vi "PositionerCapture2.vi"() -> ()   [LabVIEW 2011]
doc: "CONEX - CC Virtual Front Panel:\n\nThis is a sample of an application that can be built with the LabVIEW drivers.\n\nPress HOME / ENABLE in top left of panel to put stage in Ready state for motion."
uses:
  <vilib>/userDefined/High Color/IMAQdx.ctl
  <vilib>/Platform/TimedLoop/XDataNode/timing_clust.ctl
  <vilib>/Platform/TimedLoop/XDataNode/nitl_modes.ctl
  <vilib>/Platform/TimedLoop/XDataNode/wakeup.ctl
  <vilib>/Platform/TimedLoop/XDataNode/XDataNode.xnode
  <vilib>/Platform/TimedLoop/XDataNode/XDNodeRunTimeDep.lvlib
  <vilib>/vision/driver/NI_Vision_Acquisition_Software.lvlib
panel:
  in  "component":bool
  out "amp pos":dbl
  out "Phase":bool
  out "Amp":bool
  in  "Next":bool
  out "Current noUnits":dbl caption="mm" format="%#_6f"
  in  "lambda":dbl caption="nm" format="%#_6f"
  in  "Units":string(combo)="mm"
  in  "Go0":bool
  in  "Zero position":dbl caption="mm" format="%#_6f"
  in  "Tare":bool
  out "Relative position":dbl caption="mm" format="%#_6f"
  in  "Path to save the captures":path
  out "Image":T1(plugin-control)
  in  "(1) Go to:":dbl=1.0 caption="mm"
  out "Title":string
  in  "Set Max":bool
  in  "Set Min":bool
  in  "Max":dbl
  in  "Min":dbl
  in  "Set velocity":bool
  out "Stop cycle":bool=TRUE
  out "Title 2":string
  in  "Cycle":bool
  in  "Go2":bool
  in  "Go1":bool
  in  "(2) Go to:":dbl=1.0 caption="mm"
  in  "-":bool
  in  "+":bool
  in  "Step:":dbl caption="mm" format="%#_6f"
  out "Position History":dbl(graph)=1.5
  in  "Action":bool
  out "Stop polling":bool=TRUE
  out "Controller state description":string="STATUS"
  out "Velocity MAX":dbl=0.4
  out "Controller state":string="33"
  out "Positioner error":string="0000"
  in  "Velocity:":dbl format="%#_6f"
  in  "Exit":bool=TRUE
  out "Target position":dbl
  in  "Exit":bool
  in  "Position glissière":cluster{dbl, dbl}(slide) scale=0.0..25.0
  out "Current position":dbl caption="mm" format="%#_6f"
  # "Take an image with \"Curr. Pos\" and a label as the name.\nThe label alternates between two states.\nThe position increase an step when Amp. and Phase\nis captured for both components."
  # "mm/s"
  # "mm"
  # "Limits:"
  # "mm"
  # "(1)"
  # "(2)"
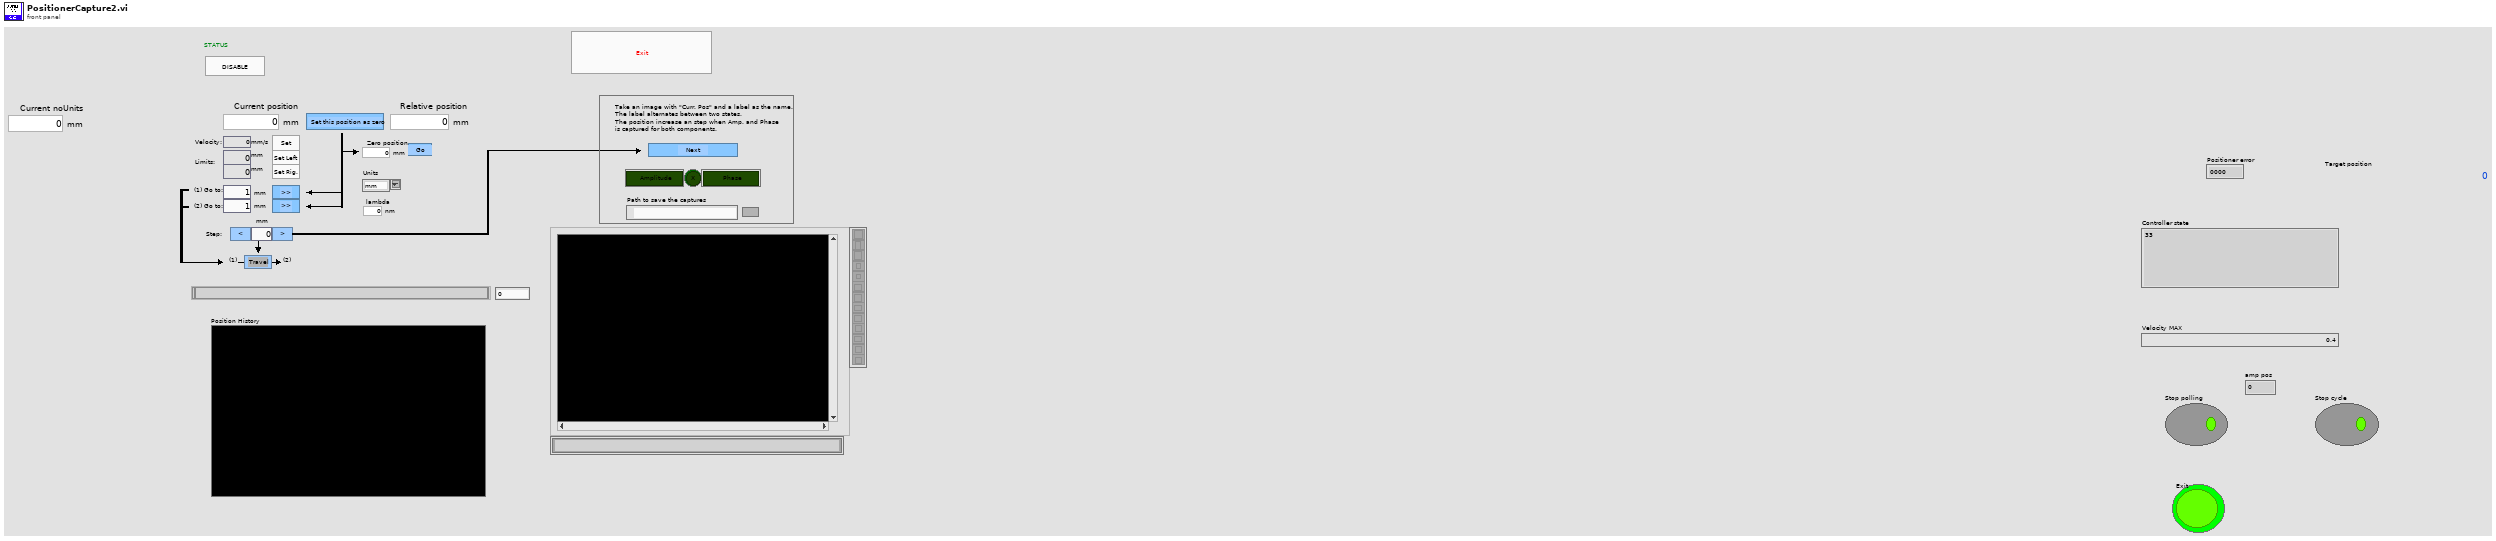
[diagram p1: front panel]
types:
  T1 = typedef "IMAQ Image.ctl" = refnum<image>
  T2 = typedef "IMAQdx.ctl" = refnum<k21>
  T3 = typedef "XDNodeRunTimeDep.lvlib/timing_clust.ctl" = cluster{"Expected End [f-1]":u64, "Actual End [f-1]":u64, "Finished Late? [f-1]":bool, "Expected End [i-1]":u64, "Actual End [i-1]":u64, "Finished Late? [i-1]":bool, "Expected Start [i]":u64, "Actual Start [i]":u64, "Expected Start [f]":u64, "Actual Start [f]":u64, "Source Name":string, "Structure Name":string, "Period":i64, "Deadline":i64, "Offset":i64, "Start":i64, "Priority":i32, "Timeout":i32, "Mode":T4, "Wakeup Reason":T5, "Error":errorcluster, "Source Type":string, "Secondary Source Type":string, "Global End Time":u64, "Global Start Time":u64, "Frame Duration":u64, "Iteration Duration":u64, "Assigned CPU":i32, "I/O Scan Engine Mode":u32}
  T4 = typedef "XDNodeRunTimeDep.lvlib/nitl_modes.ctl" = enum32{"No Change", "Process missed periods, maintain original phase", "Discard missed periods, maintain original phase", "Process missed periods, ignore original phase", "Discard missed periods, ignore original phase"}
  T5 = typedef "XDNodeRunTimeDep.lvlib/wakeup.ctl" = enum32{"Normal", "Aborted", "Asynchronous wakeup", "Timing source error", "Timed loop error", "Timeout"}
  T6 = cluster{"VISA resource name":refnum<visa-resource-name>, "Device name":string, "Controller address":i32, "error":errorcluster}
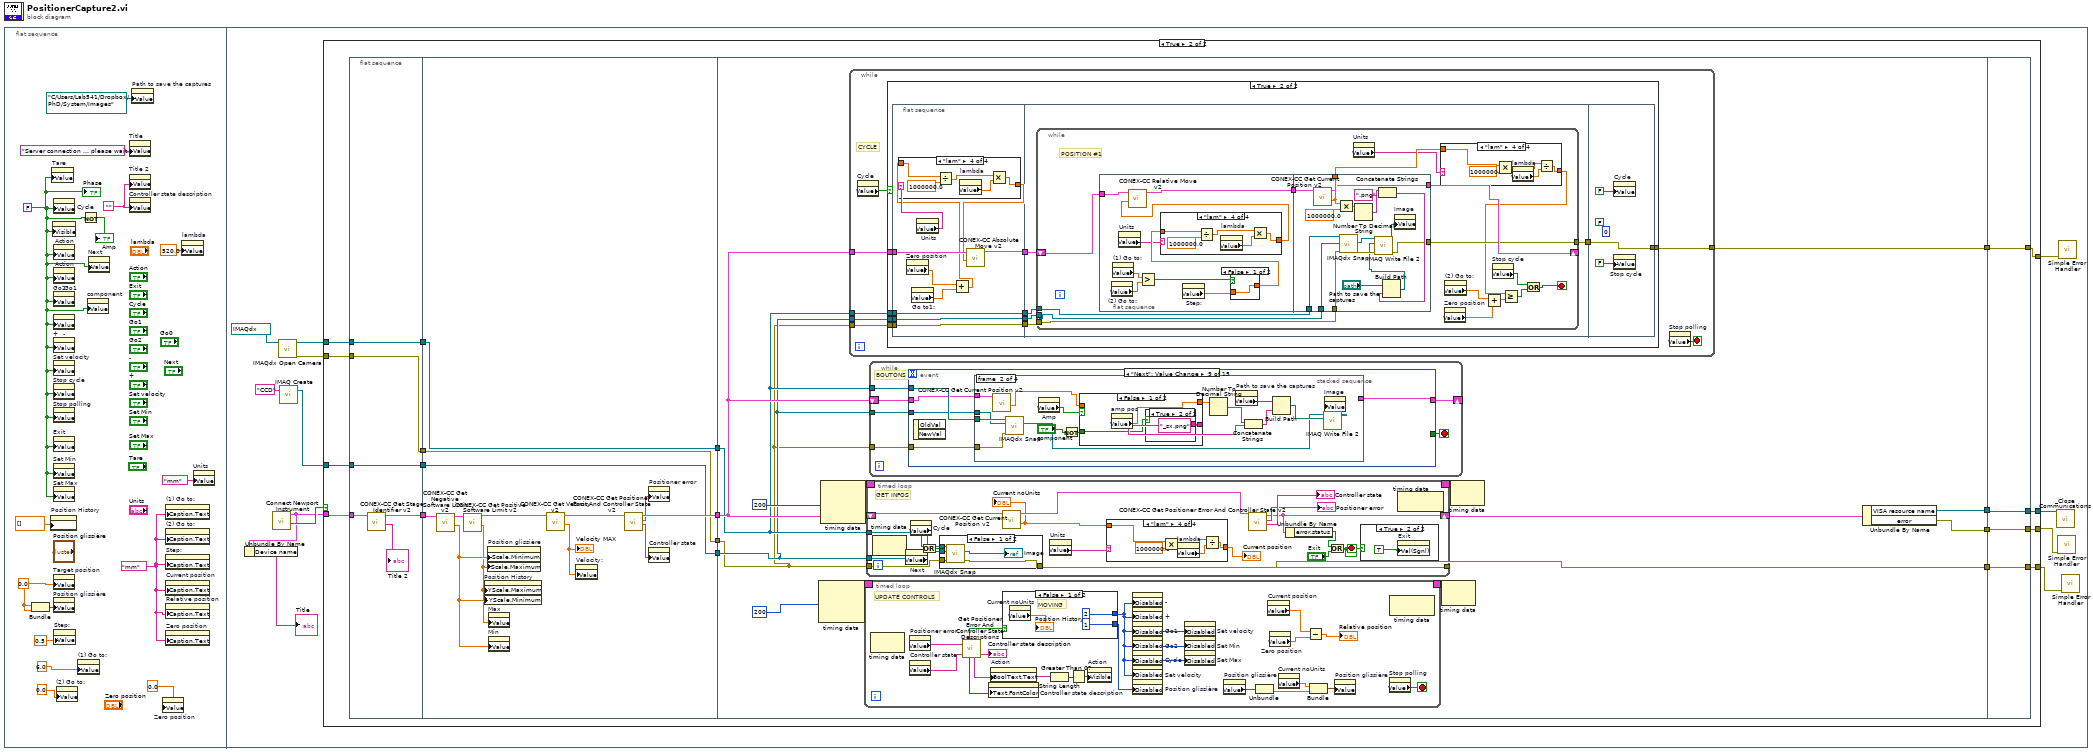
[diagram p0: block diagram]
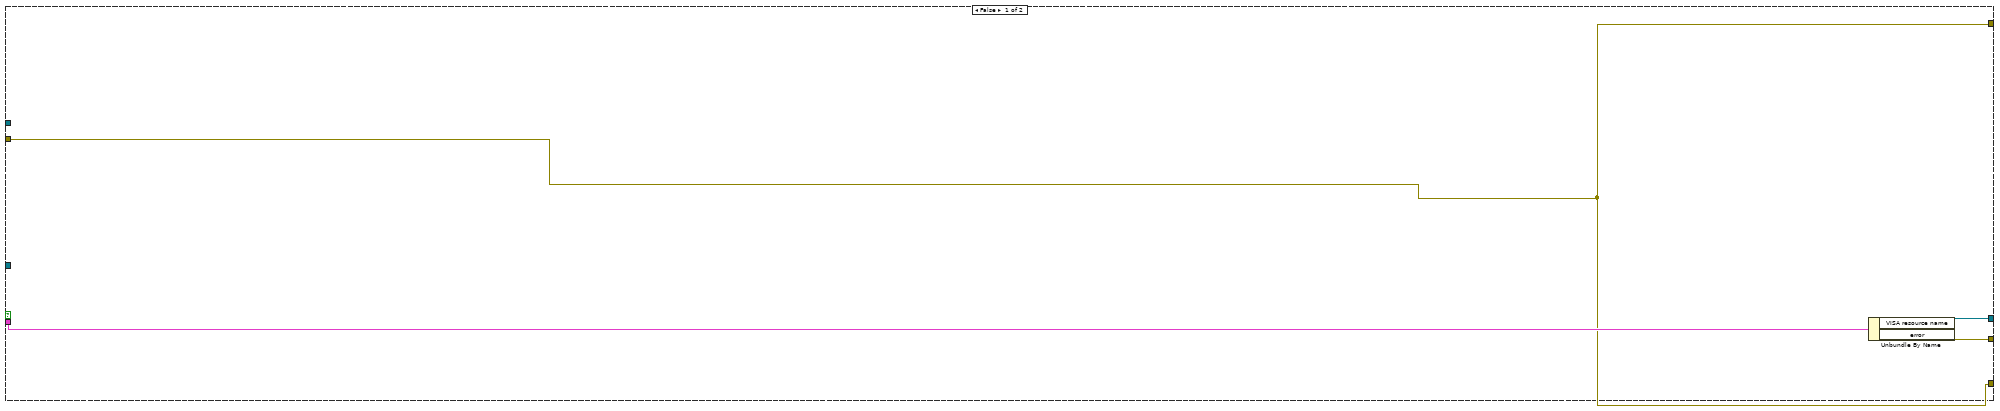
[diagram p2: hidden frame]
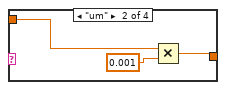
[diagram p5: hidden frame]
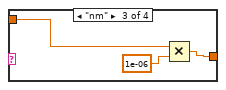
[diagram p6: hidden frame]
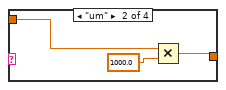
[diagram p8: hidden frame]
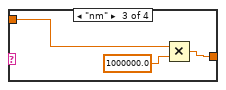
[diagram p9: hidden frame]
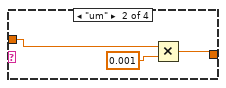
[diagram p11: hidden frame]
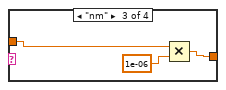
[diagram p12: hidden frame]
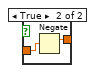
[diagram p13: hidden frame]
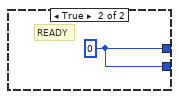
[diagram p14: hidden frame]
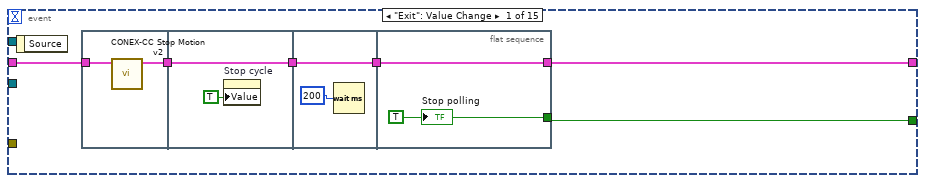
[diagram p15: hidden frame]
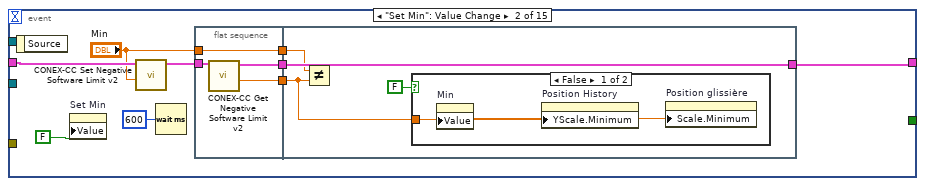
[diagram p16: hidden frame]
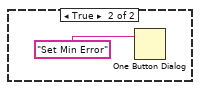
[diagram p17: hidden frame]
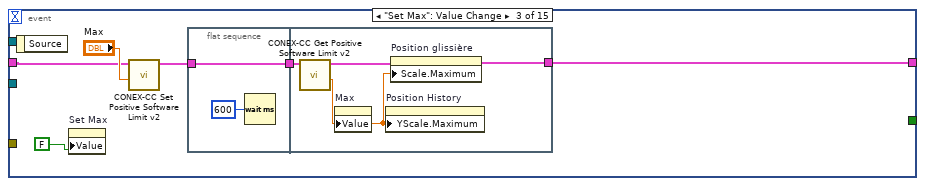
[diagram p18: hidden frame]
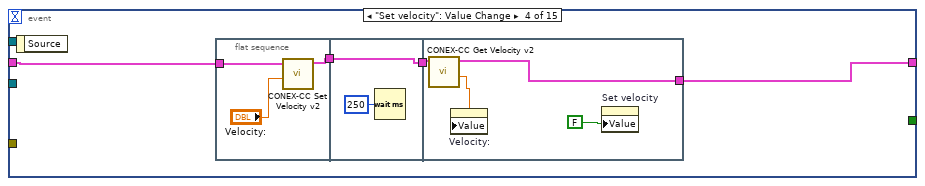
[diagram p19: hidden frame]
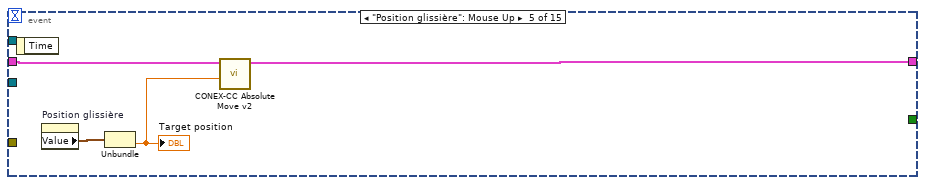
[diagram p20: hidden frame]
diagram:
  n1 = flat-sequence {
    frame #0 {
      w5 = "mm" ("Units")
      w1 = FALSE
      w14 = 0.0
      w13 = ""
      n2 = Bundle(w14, w14) -> (w15:cluster{dbl, dbl})  [unwired: 1 out]
      n3 = property on="Position History" class="WFChart (strict)"("History Data"=dbl[] [] ("Données d'historique")) -> ()  [unwired: 2 in, 2 out]
      n4 = property on="Tare" class="Bool (strict)"("Value"=w1) -> ()  [unwired: 2 in, 2 out]
      n5 = property on="Action" class="Bool (strict)"("Visible"=w1) -> ()  [unwired: 2 in, 2 out]
      n6 = property on="Cycle" class="Bool (strict)"("Value"=w1) -> ()  [unwired: 2 in, 2 out]
      n7 = property on="Action" class="Bool (strict)"("Value"=w1) -> ()  [unwired: 2 in, 2 out]
      n8 = property on="Go1" class="Bool (strict)"("Value"=w1) -> ()  [unwired: 2 in, 2 out]
      n9 = property on="Go2" class="Bool (strict)"("Value"=w1) -> ()  [unwired: 2 in, 2 out]
      n10 = property on="-" class="Bool (strict)"("Value"=w1) -> ()  [unwired: 2 in, 2 out]
      n11 = property on="+" class="Bool (strict)"("Value"=w1) -> ()  [unwired: 2 in, 2 out]
      n12 = property on="Set velocity" class="Bool (strict)"("Value"=w1) -> ()  [unwired: 2 in, 2 out]
      n13 = property on="Stop cycle" class="Bool (strict)"("Value"=w1) -> ()  [unwired: 2 in, 2 out]
      n14 = property on="Stop polling" class="Bool (strict)"("Value"=w1) -> ()  [unwired: 2 in, 2 out]
      n15 = property on="Exit" class="Bool (strict)"("Value"=w1) -> ()  [unwired: 2 in, 2 out]
      n16 = property on="Set Min" class="Bool (strict)"("Value"=w1) -> ()  [unwired: 2 in, 2 out]
      n17 = property on="Set Max" class="Bool (strict)"("Value"=w1) -> ()  [unwired: 2 in, 2 out]
      n18 = property on="Target position" class="DigNum (strict)"("Value"=w14) -> ()  [unwired: 2 in, 2 out]
      n19 = property on="Position glissière" class="Slide (strict)"("Value"=w15) -> ()  [unwired: 2 in, 2 out]
      n20 = property on="Step:" class="DigNum (strict)"("Value"=0.5 ("Step")) -> ()  [unwired: 2 in, 2 out]
      n21 = property on="(2) Go to:" class="DigNum (strict)"("Value"=0.0 ("Abs. Move 2")) -> ()  [unwired: 2 in, 2 out]
      n22 = property on="(1) Go to:" class="DigNum (strict)"("Value"=6.0 ("Abs. Move 1")) -> ()  [unwired: 2 in, 2 out]
      n23 = Not(x=w1) -> (.not. x?=→"Amp":bool)
      n24 = property on="component" class="Bool (strict)"("Value"=w1) -> ()  [unwired: 2 in, 2 out]
      n25 = property on="Next" class="Bool (strict)"("Value"=w1) -> ()  [unwired: 2 in, 2 out]
      n26 = property on="Title" class="Str"("Value"="Server connection ... please wait." ("Title")) -> ()  [unwired: 2 in, 2 out]
      n27 = property on="Title 2" class="Str"("Value"=w13) -> ()  [unwired: 2 in, 2 out]
      n28 = property on="Controller state description" class="Str"("Value"=w13) -> ()  [unwired: 2 in, 2 out]
      n29 = property on="Path to save the captures" class="Path"("Value"=path "C:/Users/Lab541/Dropbox/PhD/System/Images" ("Path to save the captures")) -> ()  [unwired: 2 in, 2 out]
      n30 = property on="Zero position" class="DigNum (strict)"("Value"=0.0 ("Zero position")) -> ()  [unwired: 2 in, 2 out]
      n31 = property on="(1) Go to:" class="DigNum (strict)"("Caption.Text"=w5) -> ()  [unwired: 2 in, 2 out]
      n32 = property on="(2) Go to:" class="DigNum (strict)"("Caption.Text"=w5) -> ()  [unwired: 2 in, 2 out]
      n33 = property on="Step:" class="DigNum (strict)"("Caption.Text"=w5) -> ()  [unwired: 2 in, 2 out]
      n34 = property on="Current position" class="DigNum (strict)"("Caption.Text"=w5) -> ()  [unwired: 2 in, 2 out]
      n35 = property on="Relative position" class="DigNum (strict)"("Caption.Text"=w5) -> ()  [unwired: 2 in, 2 out]
      n36 = property on="Zero position" class="DigNum (strict)"("Caption.Text"=w5) -> ()  [unwired: 2 in, 2 out]
      n37 = property on="lambda" class="DigNum (strict)"("Value"=520.0 ("lambda")) -> ()  [unwired: 2 in, 2 out]
      n38 = property on="Units" class="CmbBox"("Value"="mm" ("Units")) -> ()  [unwired: 2 in, 2 out]
      "Phase" <- w1
    }
    frame #1 {
      n39 = call <userlib>:"Connect Newport Instrument.vi"() -> ("Connected"=w25:bool, "Device Connection Cluster"=w24:T6)  [unwired: 7 in, 3 out]
      n40 = Unbundle By Name(w24) -> ("Device name"=→"Title":string)
      n41 = call <vilib>:"IMAQdx Open Camera.vi"("Session In"=T2 "Paraxial") -> ("error out"=w18:errorcluster, "Session Out"=w20:T2)  [unwired: 9 in]
      n42 = call "IMAQ Create"("Image Name"="CCD") -> ("New Image"=w19:T1)  [unwired: 4 in, 1 out]
      n43 = case shown="True" w25 {
        tunnel: [w30 w51] -> w27
        tunnel: w24 -> [w31 w49]
        tunnel: [w29 w45] -> w23
        tunnel: w20 -> [_ w43]
        tunnel: w19 -> [_ w40]
        tunnel: w18 -> [w28 w37]
        tunnel: [w28 w34] -> w17
        tunnel: [w28 w32] -> w16
        frame False {
          n44 = Unbundle By Name(w31) -> ("VISA resource name"=w29:refnum<visa-resource-name>, "error"=w30:errorcluster)
        }
        frame True {
          n45 = flat-sequence {
            tunnel: w49 -> [w57]
            tunnel: [w55] -> w48
            tunnel: [w54] -> w44
            tunnel: w43 -> [w54]
            tunnel: [w53] -> w41
            tunnel: w40 -> [w53]
            tunnel: [w52] -> w38
            tunnel: w37 -> [w52]
            tunnel: [w67] -> w50
            tunnel: w48 -> [w64]
            tunnel: w44 -> [w60]
            tunnel: [w60] -> w42
            tunnel: w41 -> [w59]
            tunnel: [w59] -> w39
            tunnel: w38 -> [w58]
            tunnel: [w58] -> w36
            tunnel: w50 -> [w76]
            tunnel: [w78] -> w47
            tunnel: [w77] -> w46
            tunnel: w42 -> [w73]
            tunnel: w39 -> [w72]
            tunnel: w36 -> [w71]
            tunnel: [w75] -> w35
            tunnel: [w74] -> w33
            tunnel: [w543] -> w51
            tunnel: w47 -> [w542]
            tunnel: w46 -> [w543]
            tunnel: [w542] -> w45
            tunnel: [w541] -> w34
            tunnel: w35 -> [w541]
            tunnel: [w540] -> w32
            tunnel: w33 -> [w540]
            frame #0 {
              n46 = call <userlib>:"CONEX-CC Get Stage Identifier v2.vi"("Connection Cluster in"=w57) -> ("Identifier"=→"Title 2":string, "Connection Cluster out"=w55:T6)  [unwired: 9 in]
            }
            frame #1 {
              n47 = call <userlib>:"CONEX-CC Get Negative Software Limit v2.vi"("Connection Cluster in"=w64) -> ("Left limit"=w69:dbl, "Connection Cluster out"=w63:T6)  [unwired: 9 in]
              n48 = call <userlib>:"CONEX-CC Get Positive Software Limit v2.vi"("Connection Cluster in"=w63) -> ("Right limit"=w68:dbl, "Connection Cluster out"=w62:T6)  [unwired: 9 in]
              n49 = property on="Position History" class="WFChart (strict)"("YScale.Maximum"=w68, "YScale.Minimum"=w69) -> ()  [unwired: 2 in, 2 out]
              n50 = property on="Position glissière" class="Slide (strict)"("Scale.Minimum"=w69, "Scale.Maximum"=w68) -> ()  [unwired: 2 in, 2 out]
              n51 = property on="Max" class="DigNum (strict)"("Value"=w68) -> ()  [unwired: 2 in, 2 out]
              n52 = property on="Min" class="DigNum (strict)"("Value"=w69) -> ()  [unwired: 2 in, 2 out]
              n53 = call <userlib>:"CONEX-CC Get Velocity v2.vi"("Connection Cluster in"=w62) -> ("Velocity"=w70:dbl, "Connection Cluster out"=w61:T6)  [unwired: 8 in, 1 out]
              "Velocity MAX" <- w70
              n54 = property on="Velocity:" class="DigNum (strict)"("Value"=w70) -> ()  [unwired: 2 in, 2 out]
              n55 = call <userlib>:"CONEX-CC Get Positioner Error And Controller State v2.vi"("Connection Cluster in"=w61) -> ("Controller state"=w65:string, "Positioner error"=w66:string, "Connection Cluster out"=w67:T6)  [unwired: 8 in]
              n56 = property on="Positioner error" class="Str"("Value"=w66) -> ()  [unwired: 2 in, 2 out]
              n57 = property on="Controller state" class="Str"("Value"=w65) -> ()  [unwired: 2 in, 2 out]
            }
            frame #2 {
              n58 = node-c288(i64 200 ("Période")) -> (w83:T3)  [unwired: 1 in, 1 out]
              n59 = node-c288(i64 200 ("Période")) -> (w85:T3)  [unwired: 1 in, 1 out]
              n60 = while {
                tunnel: w76 -> [w92]
                tunnel: w73 -> [w89]
                tunnel: w72 -> [w88]
                tunnel: w71 -> [w87]
                tunnel: [w86] -> w74
                stop <- w91 stop-if-true
                # "CYCLE"
                n61 = property on="Cycle" class="Bool (strict)"() -> ("Value"=w90:bool)  [unwired: 2 in, 2 out]
                n62 = case shown="True" w90 {
                  tunnel: w92 -> [_ w103]
                  tunnel: w89 -> [_ w100]
                  tunnel: w88 -> [_ w98]
                  tunnel: w87 -> [w93 w96]
                  tunnel: [w93 w95] -> w86
                  frame False {
                  }
                  frame True {
                    n63 = flat-sequence {
                      tunnel: w103 -> [w113]
                      tunnel: [w112] -> w102
                      tunnel: [w111] -> w101
                      tunnel: w100 -> [w111]
                      tunnel: [w110] -> w99
                      tunnel: w98 -> [w110]
                      tunnel: [w109] -> w97
                      tunnel: w96 -> [w109]
                      tunnel: w102 -> [w130]
                      tunnel: w101 -> [w129]
                      tunnel: w99 -> [w128]
                      tunnel: w97 -> [w127]
                      tunnel: [w126] -> w94
                      tunnel: [w200] -> w95
                      tunnel: w94 -> [w200]
                      frame #0 {
                        n64 = property on="Zero position" class="DigNum (strict)"() -> ("Value"=w104:dbl)  [unwired: 2 in, 2 out]
                        n65 = property on="Go to1:" class="DigNum (strict)"() -> ("Value"=w106:dbl)  [unwired: 2 in, 2 out]
                        n66 = property on="Units" class="CmbBox"() -> ("Value"=w107:string)  [unwired: 2 in, 2 out]
                        n67 = Add(x=w104, y=w106) -> (x+y=w105:dbl)
                        n68 = case shown="\"lam\"" w107 {
                          tunnel: [w114 w115 w118 w121] -> w108
                          tunnel: w105 -> [w114 w116 w119 w125]
                          frame "mm", Default {
                          }
                          frame "um" {
                            n69 = Multiply(x=w116, y=0.001) -> (x*y=w115:dbl)
                          }
                          frame "nm" {
                            n70 = Multiply(x=w119, y=1e-06) -> (x*y=w118:dbl)
                          }
                          frame "lam" {
                            n71 = Divide(x=w125, y=1000000.0) -> (x/y=w123:dbl)
                            n72 = property on="lambda" class="DigNum (strict)"() -> ("Value"=w122:dbl)  [unwired: 2 in, 2 out]
                            n73 = Multiply(x=w123, y=w122) -> (x*y=w121:dbl)
                          }
                        }
                        n74 = call <userlib>:"CONEX-CC Absolute Move v2.vi"("Target position"=w108, "Connection Cluster in"=w113) -> ("Connection Cluster out"=w112:T6)  [unwired: 5 in, 2 out]
                      }
                      frame #1 {
                        n75 = while {
                          shift-right: [w139] -> _
                          shift-left: w130 -> [w145]
                          tunnel: w129 -> [w141]
                          tunnel: w128 -> [w140]
                          tunnel: w127 -> [w142]
                          tunnel: [w138] -> w126
                          stop <- w146 stop-if-true
                          # "POSITION #1"
                          n76 = flat-sequence {
                            tunnel: w145 -> [w167]
                            tunnel: [w166] -> w137
                            tunnel: w141 -> [w199]
                            tunnel: w140 -> [w198]
                            tunnel: w142 -> [w197]
                            tunnel: w137 -> [w193]
                            tunnel: [w185] -> w136
                            tunnel: [w184] -> w139
                            tunnel: [w183] -> w138
                            frame #0 {
                              n77 = property on="(2) Go to:" class="DigNum (strict)"() -> ("Value"=w165:dbl)  [unwired: 2 in, 2 out]
                              n78 = property on="(1) Go to:" class="DigNum (strict)"() -> ("Value"=w164:dbl)  [unwired: 2 in, 2 out]
                              n79 = property on="Units" class="CmbBox"() -> ("Value"=w159:string)  [unwired: 2 in, 2 out]
                              n80 = Greater?(x=w164, y=w165) -> (0:w163:bool)
                              n81 = property on="Step:" class="DigNum (strict)"() -> ("Value"=w162:dbl)  [unwired: 2 in, 2 out]
                              n82 = case shown="False" w163 {
                                tunnel: [w180 w181] -> w161
                                tunnel: w162 -> [w180 w182]
                                frame False {
                                }
                                frame True {
                                n83 = Negate(x=w182) -> (-x=w181:dbl)
                                }
                              }
                              n84 = case shown="\"lam\"" w159 {
                                tunnel: [w168 w170 w173 w176] -> w160
                                tunnel: w161 -> [w168 w169 w172 w175]
                                frame "mm", Default {
                                }
                                frame "um" {
                                n85 = Multiply(x=w169, y=0.001) -> (x*y=w170:dbl)
                                }
                                frame "nm" {
                                n86 = Multiply(x=w172, y=1e-06) -> (x*y=w173:dbl)
                                }
                                frame "lam" {
                                n87 = Divide(x=w175, y=1000000.0) -> (x/y=w178:dbl)
                                n88 = property on="lambda" class="DigNum (strict)"() -> ("Value"=w177:dbl)  [unwired: 2 in, 2 out]
                                n89 = Multiply(x=w178, y=w177) -> (x*y=w176:dbl)
                                }
                              }
                              n90 = call <userlib>:"CONEX-CC Relative Move v2.vi"("Relative displacement"=w160, "Connection Cluster in"=w167) -> ("Connection Cluster out"=w166:T6)  [unwired: 9 in]
                            }
                            frame #1 {
                              n91 = call <userlib>:"CONEX-CC Get Current Position v2.vi"("Connection Cluster in"=w193) -> ("Current position"=w185:dbl, "Connection Cluster out"=w184:T6)  [unwired: 8 in, 1 out]
                              n92 = Multiply(x=w185, y=1000000.0) -> (x*y=w189:dbl)
                              n93 = call <vilib>:"IMAQdx Snap.vi"("error in"=w197, "Image In"=w198, "Session In"=w199) -> ("error out"=w195:errorcluster, "Image Out"=w196:T1)  [unwired: 6 in, 1 out]
                              n94 = Number To Decimal String(number=w189) -> (decimal integer string=w188:string)  [unwired: 1 in]
                              n95 = Concatenate Strings(w188, ".png" ("string")) -> (w186:string)
                              n96 = Build Path(base path="Path to save the captures", name or relative path=w186) -> (appended path=w190:path)
                              n97 = call-poly "IMAQ Write File 2"("error in (no error)"=w195, "File Path"=w190, "Image"=w196) -> ("error out"=w183:errorcluster, "Image Out (duplicate)"=w194:T1)  [unwired: 7 in]
                              n98 = property on="Image" class="ImageControl"("Value"=w194) -> ()  [unwired: 2 in, 2 out]
                            }
                          }
                          n99 = property on="Units" class="CmbBox"() -> ("Value"=w134:string)  [unwired: 2 in, 2 out]
                          n100 = case shown="\"lam\"" w134 {
                            tunnel: [w147 w148 w151 w154] -> w135
                            tunnel: w136 -> [w147 w149 w152 w155]
                            frame "mm", Default {
                            }
                            frame "um" {
                              n101 = Multiply(x=w149, y=1000.0) -> (x*y=w148:dbl)
                            }
                            frame "nm" {
                              n102 = Multiply(x=w152, y=1000000.0) -> (x*y=w151:dbl)
                            }
                            frame "lam" {
                              n103 = Multiply(x=w155, y=1000000.0) -> (x*y=w158:dbl)
                              n104 = property on="lambda" class="DigNum (strict)"() -> ("Value"=w156:dbl)  [unwired: 2 in, 2 out]
                              n105 = Divide(x=w158, y=w156) -> (x/y=w154:dbl)
                            }
                          }
                          n106 = property on="Zero position" class="DigNum (strict)"() -> ("Value"=w131:dbl)  [unwired: 2 in, 2 out]
                          n107 = property on="(2) Go to:" class="DigNum (strict)"() -> ("Value"=w132:dbl)  [unwired: 2 in, 2 out]
                          n108 = Add(x=w132, y=w131) -> (x+y=w133:dbl)
                          n109 = property on="Stop cycle" class="Bool (strict)"() -> ("Value"=w143:bool)  [unwired: 2 in, 2 out]
                          n110 = Greater Or Equal?(x=w135, y=w133) -> (x >= y?=w144:bool)
                          n111 = Or(x=w143, y=w144) -> (x .or. y?=w146:bool)
                        }
                      }
                      frame #2 {
                        (unwired) 0 ("counter")
                        (unwired) FALSE ("Visible")
                        n112 = property on="Cycle" class="Bool (strict)"("Value"=FALSE ("Cycle")) -> ()  [unwired: 2 in, 2 out]
                        n113 = property on="Stop cycle" class="Bool (strict)"("Value"=FALSE ("Cycle")) -> ()  [unwired: 2 in, 2 out]
                      }
                    }
                  }
                }
                n114 = property on="Stop polling" class="Bool (strict)"() -> ("Value"=w91:bool)  [unwired: 2 in, 2 out]
              }
              n115 = timed-loop {
                timing: w83 -> [_]
                timing-out: [_] -> w82
                stop <- w211 stop-if-true
                # "UPDATE CONTROLS"
                n116 = node-c288() -> ()  [unwired: 2 out]
                n117 = property on="Positioner error" class="Str"() -> ("Value"=w220:string)  [unwired: 2 in, 2 out]
                n118 = property on="Controller state" class="Str"() -> ("Value"=w219:string)  [unwired: 2 in, 2 out]
                n119 = call <userlib>:"Get Positioner Error And Controller State Descriptions.vi"("Controller state"=w219, "Positioner error"=w220) -> ("Color"=w217:u32, "Action name"=w216:string, "Controller state description"=→"Controller state description":string, "IsReady?"=w213:bool)  [unwired: 2 out]
                n120 = property on="Controller state description" class="Str"("Text.FontColor"=w217) -> ()  [unwired: 2 in, 2 out]
                n121 = property on="Action" class="Bool (strict)"("BoolText.Text"=w216) -> ()  [unwired: 2 in, 2 out]
                n122 = case shown="False" w213 {
                  tunnel: [u8 2 w224] -> w210
                  tunnel: [u8 1 w224] -> w212
                  frame False {
                    # "MOVING"
                    n123 = property on="Current noUnits" class="DigNum (strict)"() -> ("Value"=→"Position History":dbl)  [unwired: 2 in, 2 out]
                  }
                  frame True {
                    w224 = u8 0
                    # "READY"
                  }
                }
                n124 = String Length(string=w216) -> (length=w215:i32)
                n125 = Greater Than 0?(x=w215) -> (x > 0?=w214:bool)
                n126 = property on="Action" class="Bool (strict)"("Visible"=w214) -> ()  [unwired: 2 in, 2 out]
                n127 = property on="-" class="Bool (strict)"("Disabled"=w210) -> ()  [unwired: 2 in, 2 out]
                n128 = property on="+" class="Bool (strict)"("Disabled"=w210) -> ()  [unwired: 2 in, 2 out]
                n129 = property on="Go1" class="Bool (strict)"("Disabled"=w210) -> ()  [unwired: 2 in, 2 out]
                n130 = property on="Go2" class="Bool (strict)"("Disabled"=w210) -> ()  [unwired: 2 in, 2 out]
                n131 = property on="Cycle" class="Bool (strict)"("Disabled"=w210) -> ()  [unwired: 2 in, 2 out]
                n132 = property on="Set velocity" class="Bool (strict)"("Disabled"=w210) -> ()  [unwired: 2 in, 2 out]
                n133 = property on="Position glissière" class="Slide (strict)"("Disabled"=w212) -> ()  [unwired: 2 in, 2 out]
                n134 = property on="Set velocity" class="Bool (strict)"("Disabled"=w210) -> ()  [unwired: 2 in, 2 out]
                n135 = property on="Set Min" class="Bool (strict)"("Disabled"=w210) -> ()  [unwired: 2 in, 2 out]
                n136 = property on="Set Max" class="Bool (strict)"("Disabled"=w210) -> ()  [unwired: 2 in, 2 out]
                n137 = property on="Position glissière" class="Slide (strict)"() -> ("Value"=w208:cluster{dbl, dbl})  [unwired: 2 in, 2 out]
                n138 = Unbundle(w208) -> (w207:dbl)  [unwired: 1 out]
                n139 = property on="Current position" class="DigNum (strict)"() -> ("Value"=w203:dbl)  [unwired: 2 in, 2 out]
                n140 = property on="Zero position" class="DigNum (strict)"() -> ("Value"=w204:dbl)  [unwired: 2 in, 2 out]
                n141 = property on="Current noUnits" class="DigNum (strict)"() -> ("Value"=w205:dbl)  [unwired: 2 in, 2 out]
                n142 = Subtract(x=w203, y=w204) -> (x-y=→"Relative position":dbl)
                n143 = Bundle("Value"=w205, w207) -> (w209:cluster{"Value":dbl, dbl})  [unwired: 1 out]
                n144 = property on="Position glissière" class="Slide (strict)"("Value"=w209) -> ()  [unwired: 2 in, 2 out]
                n145 = node-c288() -> ()  [unwired: 2 out]
                n146 = property on="Stop polling" class="Bool (strict)"() -> ("Value"=w211:bool)  [unwired: 2 in, 2 out]
              }
              n147 = timed-loop {
                timing: w85 -> [_]
                timing-out: [_] -> w84
                shift-right: [w505] -> w79
                shift-left: w76 -> [w514]
                tunnel: w73 -> [w513]
                tunnel: w72 -> [w512]
                tunnel: w71 -> [w511]
                tunnel: [w510] -> w75
                stop <- w508 stop-if-true
                # "GET INFOS"
                n148 = node-c288() -> ()  [unwired: 2 out]
                n149 = property on="Next" class="Bool (strict)"() -> ("Value"=w497:bool)  [unwired: 2 in, 2 out]
                n150 = property on="Cycle" class="Bool (strict)"() -> ("Value"=w499:bool)  [unwired: 2 in, 2 out]
                n151 = Or(x=w499, y=w497) -> (x .or. y?=w498:bool)
                n152 = case shown="False" w498 {
                  tunnel: w513 -> [w531 _]
                  tunnel: w512 -> [w530 _]
                  tunnel: w511 -> [w529 w532]
                  tunnel: [w527 w532] -> w510
                  frame False {
                    n153 = call <vilib>:"IMAQdx Snap.vi"("error in"=w529, "Image In"=w530, "Session In"=w531) -> ("error out"=w527:errorcluster, "Image Out"=→"Image":T1)  [unwired: 6 in, 1 out]
                  }
                  frame True {
                  }
                }
                n154 = call <userlib>:"CONEX-CC Get Current Position v2.vi"("Connection Cluster in"=w514) -> ("Current position"=w501:dbl, "Connection Cluster out"=w502:T6)  [unwired: 8 in, 1 out]
                "Current noUnits" <- w501
                n155 = property on="Units" class="CmbBox"() -> ("Value"=w500:string)  [unwired: 2 in, 2 out]
                n156 = case shown="\"lam\"" w500 {
                  tunnel: [w515 w516 w519 w522] -> w504
                  tunnel: w501 -> [w515 w517 w520 w523]
                  frame "mm", Default {
                  }
                  frame "um" {
                    n157 = Multiply(x=w517, y=1000.0) -> (x*y=w516:dbl)
                  }
                  frame "nm" {
                    n158 = Multiply(x=w520, y=1000000.0) -> (x*y=w519:dbl)
                  }
                  frame "lam" {
                    n159 = Multiply(x=w523, y=1000000.0) -> (x*y=w526:dbl)
                    n160 = property on="lambda" class="DigNum (strict)"() -> ("Value"=w524:dbl)  [unwired: 2 in, 2 out]
                    n161 = Divide(x=w526, y=w524) -> (x/y=w522:dbl)
                  }
                }
                "Current position" <- w504
                n162 = call <userlib>:"CONEX-CC Get Positioner Error And Controller State v2.vi"("Connection Cluster in"=w502) -> ("Controller state"=→"Controller state":string, "Positioner error"=→"Positioner error":string, "Connection Cluster out"=w505:T6)  [unwired: 8 in]
                n163 = Unbundle By Name(w505) -> ("error.status"=w503:bool)
                n164 = Or(x=w503, y="Exit") -> (x .or. y?=w508:bool)
                n165 = case shown="True" w508 {
                  frame False {
                  }
                  frame True {
                    n166 = property on="Exit" class="Bool (strict)"("Val(Sgnl)"=TRUE) -> ()  [unwired: 2 in, 2 out]
                  }
                }
                n167 = node-c288() -> ()  [unwired: 2 out]
              }
              n168 = while {
                shift-right: [w236] -> _
                shift-left: w76 -> [w235]
                tunnel: w73 -> [w233]
                tunnel: w72 -> [w232]
                tunnel: w71 -> [w231]
                stop <- w234 stop-if-true
                # "BOUTONS"
                n169 = event shown="[8] \"Next\": Value Change" {
                  selector: _ -> [_ _ _ _ _ _ _ _ _ _ _ _ _ _ _]
                  dyn-events: _ -> [_ _ _ _ _ _ _ _ _ _ _ _ _ _ _]
                  timeout: _ -> [_ _ _ _ _ _ _ _ _ _ _ _ _ _ _]
                  tunnel: [w240 _ _ _ _ _ _ _ _ _ _ _ _ _ _] -> w234
                  tunnel: w235 -> [w237 w257 w271 w284 w296 w300 w319 w340 w357 w424 w444 w461 w477 w479 w488]
                  tunnel: [w242 w256 w270 w281 w295 w299 w318 w341 w356 w423 w443 w462 w477 w479 w488] -> w236
                  tunnel: w233 -> [_ _ _ _ _ _ _ _ w359 _ _ _ _ _ _]
                  tunnel: w232 -> [_ _ _ _ _ _ _ _ w358 _ _ _ _ _ _]
                  tunnel: w231 -> [_ _ _ _ _ _ _ _ w355 _ _ _ _ _ _]
                  event "Exit": Value Change {
                    n170 = event-data() -> ()  [unwired: 2 out]
                    n171 = flat-sequence {
                      tunnel: [w244] -> w241
                      tunnel: w237 -> [w243]
                      tunnel: w241 -> [w246]
                      tunnel: [w246] -> w239
                      tunnel: w239 -> [w248]
                      tunnel: [w248] -> w238
                      tunnel: [w250] -> w242
                      tunnel: w238 -> [w250]
                      tunnel: [w249] -> w240
                      frame #0 {
                        n172 = call <userlib>:"CONEX-CC Stop Motion v2.vi"("Connection Cluster in"=w243) -> ("Connection Cluster out"=w244:T6)  [unwired: 10 in]
                      }
                      frame #1 {
                        n173 = property on="Stop cycle" class="Bool (strict)"("Value"=TRUE) -> ()  [unwired: 2 in, 2 out]
                      }
                      frame #2 {
                        n174 = Wait (ms)(milliseconds to wait=u32 200 ("attente (ms)")) -> ()  [unwired: 1 out]
                      }
                      frame #3 {
                        w249 = TRUE
                        "Stop polling" <- w249
                      }
                    }
                  }
                  event "Set Min": Value Change {
                    n175 = event-data() -> ()  [unwired: 2 out]
                    n176 = property on="Set Min" class="Bool (strict)"("Value"=FALSE ("Set Min")) -> ()  [unwired: 2 in, 2 out]
                    n177 = call <userlib>:"CONEX-CC Set Negative Software Limit v2.vi"("Negative limit (left)"="Min", "Connection Cluster in"=w257) -> ("Connection Cluster out"=w259:T6)  [unwired: 9 in]
                    n178 = Wait (ms)(milliseconds to wait=u32 600 ("attente (ms)")) -> ()  [unwired: 1 out]
                    n179 = flat-sequence {
                      tunnel: w259 -> [w263]
                      tunnel: [w262] -> w254
                      tunnel: [w261] -> w253
                      tunnel: "Min" -> [w261]
                      tunnel: [w260] -> w251
                      tunnel: [w267] -> w256
                      tunnel: w254 -> [w267]
                      tunnel: w253 -> [w266]
                      tunnel: w251 -> [w264]
                      frame #0 {
                        n180 = call <userlib>:"CONEX-CC Get Negative Software Limit v2.vi"("Connection Cluster in"=w263) -> ("Left limit"=w260:dbl, "Connection Cluster out"=w262:T6)  [unwired: 9 in]
                      }
                      frame #1 {
                        n181 = Not Equal?(x=w266, y=w264) -> ()  [unwired: 1 out]
                        n182 = case shown="False" FALSE {
                          tunnel: w264 -> [w268 _]
                          frame False {
                            n183 = property on="Min" class="DigNum (strict)"("Value"=w268) -> ()  [unwired: 2 in, 2 out]
                            n184 = property on="Position History" class="WFChart (strict)"("YScale.Minimum"=w268) -> ()  [unwired: 2 in, 2 out]
                            n185 = property on="Position glissière" class="Slide (strict)"("Scale.Minimum"=w268) -> ()  [unwired: 2 in, 2 out]
                          }
                          frame True {
                            n186 = One Button Dialog(message="Set Min Error") -> ()  [unwired: 1 in, 1 out]
                          }
                        }
                      }
                    }
                  }
                  event "Set Max": Value Change {
                    n187 = event-data() -> ()  [unwired: 2 out]
                    n188 = property on="Set Max" class="Bool (strict)"("Value"=FALSE ("Set Max")) -> ()  [unwired: 2 in, 2 out]
                    n189 = call <userlib>:"CONEX-CC Set Positive Software Limit v2.vi"("Positive limit (right)"="Max", "Connection Cluster in"=w271) -> ("Connection Cluster out"=w275:T6)  [unwired: 9 in]
                    n190 = flat-sequence {
                      tunnel: w275 -> [w277]
                      tunnel: [w277] -> w272
                      tunnel: [w280] -> w270
                      tunnel: w272 -> [w278]
                      frame #0 {
                        n191 = Wait (ms)(milliseconds to wait=u32 600 ("attente (ms)")) -> ()  [unwired: 1 out]
                      }
                      frame #1 {
                        n192 = call <userlib>:"CONEX-CC Get Positive Software Limit v2.vi"("Connection Cluster in"=w278) -> ("Right limit"=w279:dbl, "Connection Cluster out"=w280:T6)  [unwired: 9 in]
                        n193 = property on="Max" class="DigNum (strict)"("Value"=w279) -> ()  [unwired: 2 in, 2 out]
                        n194 = property on="Position History" class="WFChart (strict)"("YScale.Maximum"=w279) -> ()  [unwired: 2 in, 2 out]
                        n195 = property on="Position glissière" class="Slide (strict)"("Scale.Maximum"=w279) -> ()  [unwired: 2 in, 2 out]
                      }
                    }
                  }
                  event "Set velocity": Value Change {
                    n196 = event-data() -> ()  [unwired: 2 out]
                    n197 = flat-sequence {
                      tunnel: w284 -> [w286]
                      tunnel: [w285] -> w282
                      tunnel: [w289] -> w283
                      tunnel: w282 -> [w289]
                      tunnel: w283 -> [w293]
                      tunnel: [w292] -> w281
                      frame #0 {
                        n198 = call <userlib>:"CONEX-CC Set Velocity v2.vi"("Velocity"="Velocity:", "Connection Cluster in"=w286) -> ("Connection Cluster out"=w285:T6)  [unwired: 9 in]
                      }
                      frame #1 {
                        n199 = Wait (ms)(milliseconds to wait=u32 250 ("attente (ms)")) -> ()  [unwired: 1 out]
                      }
                      frame #2 {
                        n200 = call <userlib>:"CONEX-CC Get Velocity v2.vi"("Connection Cluster in"=w293) -> ("Velocity"=w291:dbl, "Connection Cluster out"=w292:T6)  [unwired: 8 in, 1 out]
                        n201 = property on="Velocity:" class="DigNum (strict)"("Value"=w291) -> ()  [unwired: 2 in, 2 out]
                        n202 = property on="Set velocity" class="Bool (strict)"("Value"=FALSE ("Set velocity")) -> ()  [unwired: 2 in, 2 out]
                      }
                    }
                  }
                  event "Position glissière": Mouse Up {
                    n203 = event-data() -> ()  [unwired: 2 out]
                    n204 = property on="Position glissière" class="Slide (strict)"() -> ("Value"=w297:cluster{dbl, dbl})  [unwired: 2 in, 2 out]
                    n205 = Unbundle(w297) -> (w294:dbl)  [unwired: 1 out]
                    "Target position" <- w294
                    n206 = call <userlib>:"CONEX-CC Absolute Move v2.vi"("Target position"=w294, "Connection Cluster in"=w296) -> ("Connection Cluster out"=w295:T6)  [unwired: 5 in, 2 out]
                  }
                  event "Action": Value Change {
                    n207 = event-data() -> ()  [unwired: 2 out]
                    n208 = property on="Action" class="Bool (strict)"() -> ("BoolText.Text"=w301:string)  [unwired: 2 in, 2 out]
                    n209 = case shown="\"HOME\"" w301 {
                      tunnel: w300 -> [w303 w305 w307 w313 w315]
                      tunnel: [w302 w305 w306 w312 w317] -> w299
                      frame "ENABLE" {
                        n210 = call <userlib>:"CONEX-CC Enter-Leave DISABLE State v2.vi"("Ready? (false=DISABLE true=READY)"=TRUE ("Flag (false=DISABLE true=READY)"), "Connection Cluster in"=w303) -> ("Connection Cluster out"=w302:T6)  [unwired: 7 in]
                      }
                      frame Default {
                      }
                      frame "HOME" {
                        n211 = flat-sequence {
                          tunnel: w307 -> [w310]
                          tunnel: [w309] -> w306
                          frame #0 {
                            n212 = One Button Dialog(message="The Stage will go to the 0 position. Check that the travel is clean!") -> ()  [unwired: 1 in, 1 out]
                          }
                          frame #1 {
                            n213 = call <userlib>:"CONEX-CC Home search v2.vi"("Connection Cluster in"=w310) -> ("Connection Cluster out"=w309:T6)  [unwired: 5 in, 3 out]
                          }
                        }
                      }
                      frame "DISABLE" {
                        n214 = call <userlib>:"CONEX-CC Enter-Leave DISABLE State v2.vi"("Ready? (false=DISABLE true=READY)"=FALSE ("Flag (false=DISABLE true=READY)"), "Connection Cluster in"=w313) -> ("Connection Cluster out"=w312:T6)  [unwired: 7 in]
                      }
                      frame "STOP" {
                        n215 = call <userlib>:"CONEX-CC Stop Motion v2.vi"("Connection Cluster in"=w315) -> ("Connection Cluster out"=w317:T6)  [unwired: 10 in]
                        n216 = property on="Stop cycle" class="Bool (strict)"("Value"=TRUE) -> ()  [unwired: 2 in, 2 out]
                        "Stop cycle" <- TRUE ("Stop cycle")
                      }
                    }
                    n217 = property on="Action" class="Bool (strict)"("Value"=FALSE) -> ()  [unwired: 2 in, 2 out]
                  }
                  event "-": Value Change {
                    n218 = event-data() -> ()  [unwired: 2 out]
                    n219 = property on="-" class="Bool (strict)"("Value"=FALSE ("-")) -> ()  [unwired: 2 in, 2 out]
                    n220 = Negate(x="Step:") -> (-x=w322:dbl)
                    n221 = property on="Units" class="CmbBox"() -> ("Value"=w320:string)  [unwired: 2 in, 2 out]
                    n222 = case shown="\"lam\"" w320 {
                      tunnel: [w325 w326 w329 w332] -> w321
                      tunnel: w322 -> [w325 w327 w330 w336]
                      frame "mm", Default {
                      }
                      frame "um" {
                        n223 = Multiply(x=w327, y=0.001) -> (x*y=w326:dbl)
                      }
                      frame "nm" {
                        n224 = Multiply(x=w330, y=1e-06) -> (x*y=w329:dbl)
                      }
                      frame "lam" {
                        n225 = Divide(x=w336, y=1000000.0) -> (x/y=w334:dbl)
                        n226 = property on="lambda" class="DigNum (strict)"() -> ("Value"=w333:dbl)  [unwired: 2 in, 2 out]
                        n227 = Multiply(x=w334, y=w333) -> (x*y=w332:dbl)
                      }
                    }
                    n228 = call <userlib>:"CONEX-CC Relative Move v2.vi"("Relative displacement"=w321, "Connection Cluster in"=w319) -> ("Connection Cluster out"=w318:T6)  [unwired: 9 in]
                  }
                  event "+": Value Change {
                    n229 = event-data() -> ()  [unwired: 2 out]
                    n230 = property on="+" class="Bool (strict)"("Value"=FALSE ("+")) -> ()  [unwired: 2 in, 2 out]
                    n231 = property on="Step:" class="DigNum (strict)"() -> ("Value"=w339:dbl)  [unwired: 2 in, 2 out]
                    n232 = property on="Units" class="CmbBox"() -> ("Value"=w338:string)  [unwired: 2 in, 2 out]
                    n233 = case shown="\"lam\"" w338 {
                      tunnel: [w343 w344 w347 w350] -> w337
                      tunnel: w339 -> [w343 w345 w348 w354]
                      frame "mm", Default {
                      }
                      frame "um" {
                        n234 = Multiply(x=w345, y=0.001) -> (x*y=w344:dbl)
                      }
                      frame "nm" {
                        n235 = Multiply(x=w348, y=1e-06) -> (x*y=w347:dbl)
                      }
                      frame "lam" {
                        n236 = Divide(x=w354, y=1000000.0) -> (x/y=w352:dbl)
                        n237 = property on="lambda" class="DigNum (strict)"() -> ("Value"=w351:dbl)  [unwired: 2 in, 2 out]
                        n238 = Multiply(x=w352, y=w351) -> (x*y=w350:dbl)
                      }
                    }
                    n239 = call <userlib>:"CONEX-CC Relative Move v2.vi"("Relative displacement"=w337, "Connection Cluster in"=w340) -> ("Connection Cluster out"=w341:T6)  [unwired: 9 in]
                  }
                  event "Next": Value Change {
                    n240 = event-data() -> ()  [unwired: 3 out]
                    n241 = stacked-sequence {
                      tunnel: w359 -> [_ w373 _ _]
                      tunnel: w358 -> [_ w372 _ _]
                      tunnel: w357 -> [_ w371 w394 _]
                      tunnel: [_ _ w393 _] -> w356
                      tunnel: w355 -> [_ w367 _ _]
                      frame #0 {
                        n242 = Wait (ms)(milliseconds to wait=u32 500) -> ()  [unwired: 1 out]
                      }
                      frame #1 {
                        n243 = call <userlib>:"CONEX-CC Get Current Position v2.vi"("Connection Cluster in"=w371) -> ("Current position"=w369:dbl)  [unwired: 8 in, 2 out]
                        n244 = call <vilib>:"IMAQdx Snap.vi"("error in"=w367, "Image In"=w372, "Session In"=w373) -> ("Image Out"=w366:T1)  [unwired: 6 in, 2 out]
                        n245 = property on="Amp" class="Bool (strict)"() -> ("Value"=w363:bool)  [unwired: 2 in, 2 out]
                        n246 = Not(x="component") -> (.not. x?=w361:bool)
                        n247 = case shown="False" w363 {
                          tunnel: [w379 w386] -> w375
                          tunnel: w369 -> [_ w384]
                          tunnel: [w378 w383] -> w368
                          tunnel: w361 -> [w377 w382]
                          frame False {
                            n248 = property on="amp pos" class="DigNum (strict)"() -> ("Value"=w378:dbl)  [unwired: 2 in, 2 out]
                            n249 = case shown="True" w377 {
                              tunnel: ["_sy.png" ("string") "_sx.png" ("string")] -> w379
                              frame False {
                              }
                              frame True {
                              }
                            }
                          }
                          frame True {
                            n250 = Multiply(x=w384, y=1000000.0) -> (x*y=w383:dbl)
                            "amp pos" <- w383
                            n251 = case shown="True" w382 {
                              tunnel: ["_Ay.png" ("string") "_Ax.png" ("string")] -> w386
                              frame False {
                              }
                              frame True {
                              }
                            }
                          }
                        }
                        n252 = Number To Decimal String(number=w368) -> (decimal integer string=w376:string)  [unwired: 1 in]
                        n253 = property on="Path to save the captures" class="Path"() -> ("Value"=w364:path)  [unwired: 2 in, 2 out]
                        n254 = Concatenate Strings(w376, w375) -> (w365:string)
                        n255 = Build Path(base path=w364, name or relative path=w365) -> (appended path=w374:path)
                        n256 = call-poly "IMAQ Write File 2"("File Path"=w374, "Image"=w366) -> ("Image Out (duplicate)"=w370:T1)  [unwired: 8 in, 1 out]
                        n257 = property on="Image" class="ImageControl"("Value"=w370) -> ()  [unwired: 2 in, 2 out]
                      }
                      frame #2 {
                        n258 = property on="component" class="Bool (strict)"() -> ("Value"=w392:bool)  [unwired: 2 in, 2 out]
                        n259 = property on="Amp" class="Bool (strict)"() -> ("Value"=w389:bool)  [unwired: 2 in, 2 out]
                        n260 = Not(x=w392) -> (.not. x?=w390:bool)
                        n261 = Or(x=w389, y=w390) -> (x .or. y?=w391:bool)
                        n262 = case shown="False" w391 {
                          tunnel: w394 -> [w399 w412]
                          tunnel: [w398 w412] -> w393
                          frame False {
                            n263 = property on="Step:" class="DigNum (strict)"() -> ("Value"=w396:dbl)  [unwired: 2 in, 2 out]
                            n264 = property on="Units" class="CmbBox"() -> ("Value"=w395:string)  [unwired: 2 in, 2 out]
                            n265 = case shown="\"lam\"" w395 {
                              tunnel: [w400 w402 w405 w408] -> w397
                              tunnel: w396 -> [w400 w401 w404 w407]
                              frame "mm", Default {
                              }
                              frame "um" {
                                n266 = Multiply(x=w401, y=0.001) -> (x*y=w402:dbl)
                              }
                              frame "nm" {
                                n267 = Multiply(x=w404, y=1e-06) -> (x*y=w405:dbl)
                              }
                              frame "lam" {
                                n268 = Divide(x=w407, y=1000000.0) -> (x/y=w410:dbl)
                                n269 = property on="lambda" class="DigNum (strict)"() -> ("Value"=w409:dbl)  [unwired: 2 in, 2 out]
                                n270 = Multiply(x=w410, y=w409) -> (x*y=w408:dbl)
                              }
                            }
                            n271 = call <userlib>:"CONEX-CC Relative Move v2.vi"("Relative displacement"=w397, "Connection Cluster in"=w399) -> ("Connection Cluster out"=w398:T6)  [unwired: 9 in]
                          }
                          frame True {
                          }
                        }
                      }
                      frame #3 {
                        n272 = property on="Next" class="Bool (strict)"("Value"=FALSE ("Next")) -> ()  [unwired: 2 in, 2 out]
                        n273 = property on="Amp" class="Bool (strict)"() -> ("Value"=w413:bool)  [unwired: 2 in, 2 out]
                        n274 = Not(x=w413) -> (.not. x?=w415:bool)
                        n275 = property on="Amp" class="Bool (strict)"("Value"=w415) -> ()  [unwired: 2 in, 2 out]
                        n276 = property on="Phase" class="Bool (strict)"("Value"=w413) -> ()  [unwired: 2 in, 2 out]
                        n277 = case shown="False" w413 {
                          frame False {
                            n278 = property on="component" class="Bool (strict)"() -> ("Value"=w417:bool)  [unwired: 2 in, 2 out]
                            n279 = Not(x=w417) -> (.not. x?=w416:bool)
                            n280 = property on="component" class="Bool (strict)"("Value"=w416) -> ()  [unwired: 2 in, 2 out]
                          }
                          frame True {
                          }
                        }
                      }
                    }
                  }
                  event "Go1": Value Change {
                    n281 = event-data() -> ()  [unwired: 2 out]
                    n282 = property on="Go1" class="Bool (strict)"("Value"=FALSE ("Go1")) -> ()  [unwired: 2 in, 2 out]
                    n283 = property on="Zero position" class="DigNum (strict)"() -> ("Value"=w421:dbl)  [unwired: 2 in, 2 out]
                    n284 = property on="Units" class="CmbBox"() -> ("Value"=w422:string)  [unwired: 2 in, 2 out]
                    n285 = Add(x="(1) Go to:", y=w421) -> (x+y=w419:dbl)
                    n286 = case shown="\"lam\"" w422 {
                      tunnel: [w426 w427 w430 w433] -> w418
                      tunnel: w419 -> [w426 w428 w431 w437]
                      frame "mm", Default {
                      }
                      frame "um" {
                        n287 = Multiply(x=w428, y=0.001) -> (x*y=w427:dbl)
                      }
                      frame "nm" {
                        n288 = Multiply(x=w431, y=1e-06) -> (x*y=w430:dbl)
                      }
                      frame "lam" {
                        n289 = Divide(x=w437, y=1000000.0) -> (x/y=w435:dbl)
                        n290 = property on="lambda" class="DigNum (strict)"() -> ("Value"=w434:dbl)  [unwired: 2 in, 2 out]
                        n291 = Multiply(x=w435, y=w434) -> (x*y=w433:dbl)
                      }
                    }
                    n292 = call <userlib>:"CONEX-CC Absolute Move v2.vi"("Target position"=w418, "Connection Cluster in"=w424) -> ("Connection Cluster out"=w423:T6)  [unwired: 5 in, 2 out]
                  }
                  event "Go2": Value Change {
                    n293 = event-data() -> ()  [unwired: 2 out]
                    n294 = property on="Go2" class="Bool (strict)"("Value"=FALSE ("Go2")) -> ()  [unwired: 2 in, 2 out]
                    n295 = property on="Zero position" class="DigNum (strict)"() -> ("Value"=w441:dbl)  [unwired: 2 in, 2 out]
                    n296 = property on="Units" class="CmbBox"() -> ("Value"=w442:string)  [unwired: 2 in, 2 out]
                    n297 = Add(x="(2) Go to:", y=w441) -> (x+y=w439:dbl)
                    n298 = case shown="\"lam\"" w442 {
                      tunnel: [w446 w448 w451 w454] -> w438
                      tunnel: w439 -> [w446 w447 w450 w453]
                      frame "mm", Default {
                      }
                      frame "um" {
                        n299 = Multiply(x=w447, y=0.001) -> (x*y=w448:dbl)
                      }
                      frame "nm" {
                        n300 = Multiply(x=w450, y=1e-06) -> (x*y=w451:dbl)
                      }
                      frame "lam" {
                        n301 = Divide(x=w453, y=1000000.0) -> (x/y=w456:dbl)
                        n302 = property on="lambda" class="DigNum (strict)"() -> ("Value"=w455:dbl)  [unwired: 2 in, 2 out]
                        n303 = Multiply(x=w456, y=w455) -> (x*y=w454:dbl)
                      }
                    }
                    n304 = call <userlib>:"CONEX-CC Absolute Move v2.vi"("Target position"=w438, "Connection Cluster in"=w444) -> ("Connection Cluster out"=w443:T6)  [unwired: 5 in, 2 out]
                  }
                  event "Go0": Value Change {
                    n305 = event-data() -> ()  [unwired: 2 out]
                    n306 = property on="Zero position" class="DigNum (strict)"() -> ("Value"=w458:dbl)  [unwired: 2 in, 2 out]
                    n307 = property on="Go0" class="Bool (strict)"("Value"=FALSE ("Go2")) -> ()  [unwired: 2 in, 2 out]
                    n308 = property on="Units" class="CmbBox"() -> ("Value"=w459:string)  [unwired: 2 in, 2 out]
                    n309 = case shown="\"lam\"" w459 {
                      tunnel: [w464 w466 w469 w472] -> w460
                      tunnel: w458 -> [w464 w465 w468 w471]
                      frame "mm", Default {
                      }
                      frame "um" {
                        n310 = Multiply(x=w465, y=0.001) -> (x*y=w466:dbl)
                      }
                      frame "nm" {
                        n311 = Multiply(x=w468, y=1e-06) -> (x*y=w469:dbl)
                      }
                      frame "lam" {
                        n312 = Divide(x=w471, y=1000000.0) -> (x/y=w474:dbl)
                        n313 = property on="lambda" class="DigNum (strict)"() -> ("Value"=w473:dbl)  [unwired: 2 in, 2 out]
                        n314 = Multiply(x=w474, y=w473) -> (x*y=w472:dbl)
                      }
                    }
                    n315 = call <userlib>:"CONEX-CC Absolute Move v2.vi"("Target position"=w460, "Connection Cluster in"=w461) -> ("Connection Cluster out"=w462:T6)  [unwired: 5 in, 2 out]
                  }
                  event "Tare": Value Change {
                    n316 = event-data() -> ()  [unwired: 2 out]
                    n317 = property on="Tare" class="Bool (strict)"("Value"=FALSE ("Tare")) -> ()  [unwired: 2 in, 2 out]
                    n318 = property on="Current position" class="DigNum (strict)"() -> ("Value"=w476:dbl)  [unwired: 2 in, 2 out]
                    n319 = property on="Zero position" class="DigNum (strict)"("Value"=w476) -> ()  [unwired: 2 in, 2 out]
                  }
                  event "Cycle": Value Change {
                    (unwired) 0 ("Numérique")
                    n320 = event-data() -> ()  [unwired: 2 out]
                    n321 = property on="Cycle" class="Bool (strict)"("Value"=TRUE ("Cycle")) -> ()  [unwired: 2 in, 2 out]
                  }
                  event "Units": Value Change {
                    n322 = event-data() -> ("NewVal"=w487:string, "OldVal"=w486:string)  [unwired: 1 out]
                    n323 = property on="(1) Go to:" class="DigNum (strict)"("Caption.Text"=w487) -> ()  [unwired: 2 in, 2 out]
                    n324 = property on="(2) Go to:" class="DigNum (strict)"("Caption.Text"=w487) -> ()  [unwired: 2 in, 2 out]
                    n325 = property on="Step:" class="DigNum (strict)"("Caption.Text"=w487) -> ()  [unwired: 2 in, 2 out]
                    n326 = property on="Current position" class="DigNum (strict)"("Caption.Text"=w487) -> ()  [unwired: 2 in, 2 out]
                    n327 = property on="Relative position" class="DigNum (strict)"("Caption.Text"=w487) -> ()  [unwired: 2 in, 2 out]
                    n328 = property on="Zero position" class="DigNum (strict)"("Caption.Text"=w487) -> ()  [unwired: 2 in, 2 out]
                    n329 = case shown="\"mm\", Default" w486 {
                      tunnel: [1000000.0 ("y") 1000.0 ("y") 1.0 ("y") w492] -> w485
                      frame "mm", Default {
                      }
                      frame "um" {
                      }
                      frame "nm" {
                      }
                      frame "lam" {
                        n330 = property on="lambda" class="DigNum (strict)"() -> ("Value"=w492:dbl)  [unwired: 2 in, 2 out]
                      }
                    }
                    n331 = case shown="\"lam\"" w487 {
                      tunnel: [1000000.0 ("y") 1000.0 ("y") 1.0 ("y") w496] -> w484
                      frame "mm", Default {
                      }
                      frame "um" {
                      }
                      frame "nm" {
                      }
                      frame "lam" {
                        n332 = property on="lambda" class="DigNum (strict)"() -> ("Value"=w496:dbl)  [unwired: 2 in, 2 out]
                      }
                    }
                    n333 = property on="Zero position" class="DigNum (strict)"() -> ("Value"=w482:dbl)  [unwired: 2 in, 2 out]
                    n334 = Divide(x=w485, y=w484) -> (x/y=w483:dbl)
                    n335 = Multiply(x=w482, y=w483) -> (x*y=w481:dbl)
                    n336 = property on="Zero position" class="DigNum (strict)"("Value"=w481) -> ()  [unwired: 2 in, 2 out]
                  }
                }
              }
              n337 = node-c288(w82) -> ()  [unwired: 1 out]
              n338 = node-c288(w84) -> ()  [unwired: 1 out]
              n339 = Unbundle By Name(w79) -> ("VISA resource name"=w78:refnum<visa-resource-name>, "error"=w77:errorcluster)
            }
            frame #3 {
            }
          }
        }
      }
      n340 = call <userlib>:"_Close Communications.vi"("Instrument Channel"=w23) -> ()  [unwired: 14 in, 1 out]
      n341 = call <vilib>:"Simple Error Handler.vi"("error in (no error)"=w27) -> ()  [unwired: 1 in, 8 out]
      n342 = call <vilib>:"Simple Error Handler.vi"("error in (no error)"=w16) -> ()  [unwired: 1 in, 8 out]
      n343 = call <vilib>:"Simple Error Handler.vi"("error in (no error)"=w17) -> ()  [unwired: 1 in, 8 out]
    }
  }
